vi "pthread_cond_timedwait.vi"(8 "error in (no error)":errorcluster, 9 "absolute time":cluster{"sec":u64, "nsec":u64}, 10 "mutex ptr in":u64, 11 "cond ptr in":u64) -> (0 "error out":errorcluster, 1 "timed out?":bool, 2 "mutex ptr out":u64, 3 "cond ptr out":u64)   [LabVIEW 2013, in "POSIX Threads.lvlib" / "POSIX Thread Object.lvclass"]
uses:
  POSIX Thread Object.lvclass
  Controls/pthread functions.ctl
  <vilib>/NI/NI Linux RT Errno/Controls/Public/errno.ctl
  <vilib>/NI/NI Linux RT Errno/Linux Errno.lvlib
  <vilib>/NI/NI Linux RT Utilities/Linux RT Utilities.lvlib
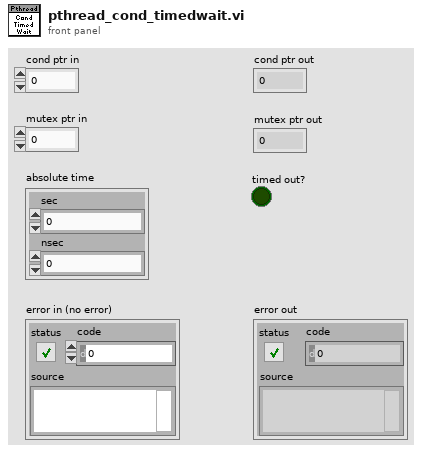
[diagram p1: front panel]
types:
  T1 = typedef "Linux Errno.lvlib/errno.ctl" = enum16{"NONE", "EPERM", "ENOENT", "ESRCH", "EINTR", "EIO", "ENXIO", "E2BIG", "ENOEXEC", "EBADF", "ECHILD", "EAGAIN", "ENOMEM", "EACCES", "EFAULT", "ENOTBLK", "EBUSY", "EEXIST", "EXDEV", "ENODEV", "ENOTDIR", "EISDIR", "EINVAL", "ENFILE", "EMFILE", "ENOTTY", "ETXTBSY", "EFBIG", "ENOSPC", "ESPIPE", "EROFS", "EMLINK", "EPIPE", "EDOM", "ERANGE", "EDADLK", "ENAMETOOLONG", "ENOLCK", "ENOSYS", "ENOTEMPTY", "ELOOP", "EWOULDBLOCK", "ENOMSG", "EIDRM", "ECHRNG", "EL2NSYNC", "EL3HLT", "EL3RST", "ELNRNG", "EUNATCH", "ENOCSI", "EL2HLT", "EBADE", "EBADR", "EXFULL", "ENOANO", "EBADRQC", "EBADSLT", "EDEADLOCK", "EBFONT", "ENOSTR", "ENODATA", "ETIME", "ENOSR", "ENONET", "ENOPKG", "EREMOTE", "ENOLINK", "EADV", "ESRMNT", "ECOMM", "EPROTO", "EMULTIHOP", "EDOTDOT", "EBADMSG", "EOVERFLOW", "ENOTUNIQ", "EBADFD", "EREMCHG", "ELIBACC", "ELIBBAD", "ELIBSCN", "ELIBMAX", "ELIBEXEC", "ELISEQ", "ERESTART", "ESTRPIPE", "EUSERS", "ENOTSOCK", "EDESTADDRREQ", "EMSGSIZE", "EPROTOTYPE", "ENOPROTOOPT", "EPROTONOSUPPORT", "ESOCKTNOSUPPORT", "EOPNOTSUPP", "EPFNOSUPPORT", "EAFNOSUPPORT", "EADDRINUSE", "EADDRNOTAVAIL", "ENETDOWN", "ENETUNREACH", "ENETRESET", "ECONNABORTED", "ECONNRESET", "ENOBUFS", "EISCONN", "ENOTCONN", "ESHUTDOWN", "ETOOMANYREFS", "ETIMEDOUT", "ECONNREFUSED", "EHOSTDOWN", "EHOSTUNREACH", "EALREADY", "EINPROGRESS", "ESTALE", "EUCLEAN", "ENOTNAM", "ENAVAIL", "EISNAM", "EREMOTEIO", "EDQUOT", "ENOMEDIUM", "EMEDIUMTYPE", "ECANCELED", "ENOKEY", "EKEYEXPIRED", "EKEYREVOKED", "EKEYREJECTED", "EOWNERDEAD", "ENOTRECOVERABLE", "ERFKILL", "EHWPOISON", "UNDEFINED"}
  T2 = typedef "POSIX Threads.lvlib/POSIX Thread Object.lvclass/pthread functions.ctl" = enum16{"unspecified", "pthread_condattr_init", "pthread_condattr_destroy", "pthread_condattr_getclock", "pthread_condattr_setclock", "pthread_condattr_getpshared", "pthread_condattr_setpshared", "pthread_cond_init", "pthread_cond_destroy", "pthread_cond_broadcast", "pthread_cond_signal", "pthread_cond_timedwait", "pthread_cond_wait", "pthread_mutexattr_init", "pthread_mutexattr_destroy", "pthread_mutexattr_getprioceiling", "pthread_mutexattr_setprioceiling", "pthread_mutexattr_getprotocol", "pthread_mutexattr_setprotocol", "pthread_mutexattr_getpshared", "pthread_mutexattr_setpshared", "pthread_mutexattr_gettype", "pthread_mutexattr_settype", "pthread_mutex_init", "pthread_mutex_destroy", "pthread_mutex_getprioceiling", "pthread_mutex_setprioceiling", "pthread_mutex_lock", "pthread_mutex_timedlock", "pthread_mutex_trylock", "pthread_mutex_unlock", "sem_destroy", "sem_getvalue", "sem_init", "sem_post", "sem_timedwait", "sem_trywait", "sem_wait", "barrier_init", "barrier_destroy", "barrier_wait", "barrierattr_init", "barrierattr_destroy", "barrierattr_getpshared", "barrierattr_setpshared"}
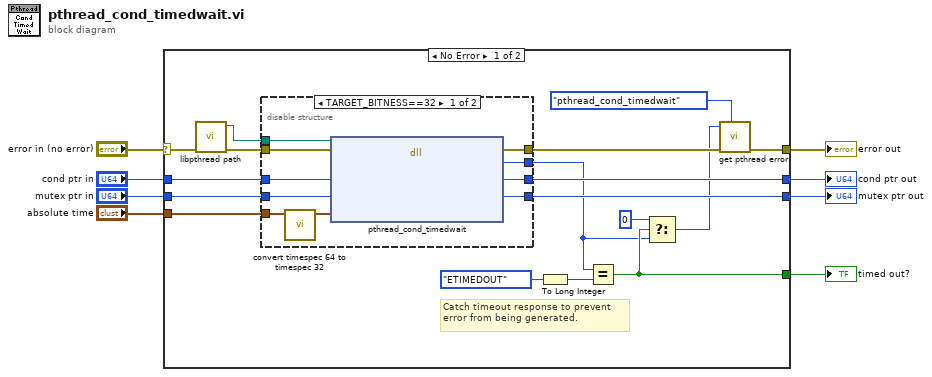
[diagram p0: block diagram]
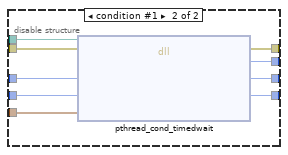
[diagram p2: hidden frame]
diagram:
  n1 = case shown="No Error" "error in (no error)" {
    selector: "error in (no error)" -> [w25 w47]
    tunnel: "cond ptr in" -> [w24 w46]
    tunnel: [w23 w47] -> w6
    tunnel: "mutex ptr in" -> [w22 w45]
    tunnel: "absolute time" -> [w21 _]
    tunnel: [w20 w46] -> w3
    tunnel: [w19 w45] -> w2
    tunnel: [w18 _] -> w1
    frame No Error {
      # "Catch timeout response to prevent error from being generated."
      n2 = call "libpthread path.vi"("error in (no error)"=w25) -> ("error out"=w17:errorcluster, "path to libpthread"=w9:path)  [unwired: 9 in]
      n3 = disable-structure shown="TARGET_BITNESS==32" {
        disable-tunnel: w24 -> [w35 w44]
        disable-tunnel: w22 -> [w34 w43]
        disable-tunnel: w21 -> [w26 w36]
        disable-tunnel: [w33 w42] -> w20
        disable-tunnel: [w32 w41] -> w19
        disable-tunnel: w17 -> [w31 w40]
        disable-tunnel: [w30 w39] -> w16
        disable-tunnel: [w29 w38] -> w12
        disable-tunnel: w9 -> [w28 w37]
        frame condition #0 (active) {
          n4 = call <vilib>:"convert timespec 64 to timespec 32.vi"("timespec 64"=w26) -> ("timespec 32"=w27:cluster{"sec":u32, "nsec":u32})  [unwired: 10 in]
          n5 = dll-call lib="?" fn="pthread_cond_timedwait"(path in=w28, error in=w31, "cond"=w35, "mutex"=w34, "abstime"=w27) -> (error out=w30:errorcluster, "errno"=w29:i32, "cond"=w33:u64, "mutex"=w32:u64)  [unwired: 2 in, 1 out]
        }
        frame condition #1 {
          n6 = dll-call lib="?" fn="pthread_cond_timedwait"(path in=w37, error in=w40, "cond"=w44, "mutex"=w43, "abstime"=w36) -> (error out=w39:errorcluster, "errno"=w38:i32, "cond"=w42:u64, "mutex"=w41:u64)  [unwired: 2 in, 1 out]
        }
      }
      n7 = To Long Integer(number=errno."ETIMEDOUT" ("errno")) -> (32bit integer=w14:i32)
      n8 = Equal?(x=w12, y=w14) -> (x = y?=w18:bool)
      n9 = Select(t=0, s=w18, f=w12) -> (s? t:f=w11:i32)
      n10 = call "get pthread error.vi"("function"=pthread_functions."pthread_cond_timedwait", "error in (no error)"=w16, "errno"=w11) -> ("error out"=w23:errorcluster)  [unwired: 8 in]
    }
    frame Error {
    }
  }
  "error out" <- w6
  "cond ptr out" <- w3
  "mutex ptr out" <- w2
  "timed out?" <- w1
